vi "Get Hardware Information.vi"(8 "error in":errorcluster, 11 "module handle in":u8) -> (0 "error out":errorcluster, 2 "hardware information":T1 {"capability_flags" format="%.0x"; "serial" format="%.0x"}, 3 "module handle out":u8)   [LabVIEW 2020, in "AIM ARINC 429 Hardware API.lvlib"]
uses:
  AIM ARINC 429 Hardware API.lvlib
  <instrlib>/_AIM 429/Session/controls/api429_board_info.ctl
  <instrlib>/_AIM 429/Session/Session.lvclass
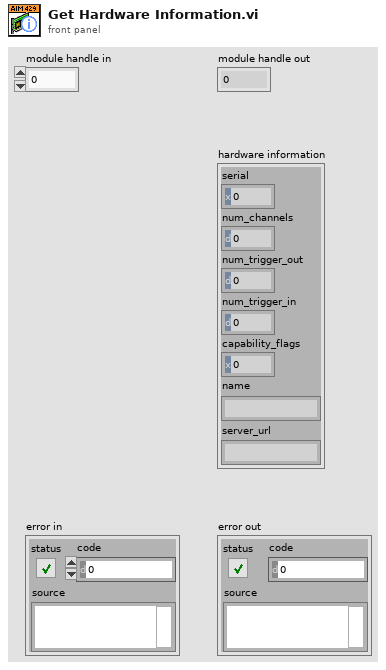
[diagram p1: front panel]
types:
  T1 = typedef "AIM429LV.lvlib/Session.lvclass/api429_board_info.ctl" = cluster{"serial":u32, "num_channels":u32, "num_trigger_out":u32, "num_trigger_in":u32, "capability_flags":u32, "name":string, "server_url":string}
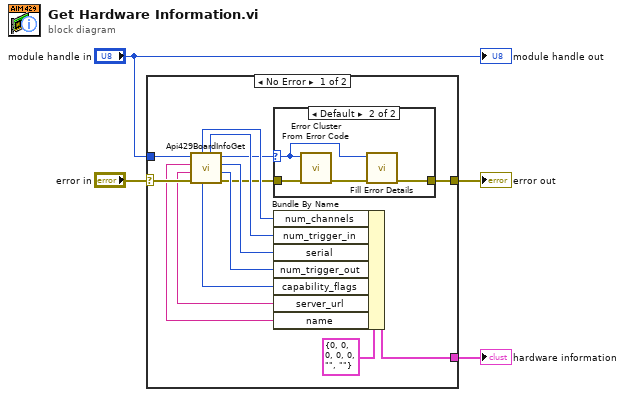
[diagram p0: block diagram]
diagram:
  n1 = case shown="No Error" "error in" {
    selector: "error in" -> [w18 w23]
    tunnel: [w5 w23] -> w2
    tunnel: [w12 _] -> w3
    tunnel: "module handle in" -> [w11 _]
    frame No Error {
      n2 = call <instrlib>:"Api429BoardInfoGet.vi"("error in (no error)"=w18, "board_handle"=w11) -> ("error out"=w6:errorcluster, "num_trigger_out"=w13:u32, "serial"=w14:u32, "error code"=w7:i32, "num_trigger_in"=w9:u32, "capability_flags"=w15:u32, "num_channels"=w10:u32, "server_url"=w16:string, "name"=w8:string)
      n3 = case shown="Default" w7 {
        selector: w7 -> [_ w22]
        tunnel: w6 -> [w19 w21]
        tunnel: [w19 w20] -> w5
        frame 0 {
        }
        frame Default {
          n4 = call <vilib>:"Error Cluster From Error Code.vi"("error in (no error)"=w21, "error code (0)"=w22) -> ()  [unwired: 7 in, 1 out]
          n5 = call "Fill Error Details.vi"("error in"=w21, "error code"=w22) -> ("error out"=w20:errorcluster)  [unwired: 9 in]
        }
      }
      n6 = Bundle By Name(cluster=T1 {"serial"=0, "num_channels"=0, "num_trigger_out"=0, "num_trigger_in"=0, "capability_flags"=0, "name"="", "server_url"=""} ("Cluster"), "num_channels"=w10, "num_trigger_in"=w9, "serial"=w14, "num_trigger_out"=w13, "capability_flags"=w15, "server_url"=w16, "name"=w8) -> (w12:T1)
    }
    frame Error {
    }
  }
  "hardware information" <- w3
  "error out" <- w2
  "module handle out" <- "module handle in"
